vi "LEBITVacuum.CreateLogFile.vi"(0 "i ref in":refnum<vi>, 2 "i attribute in":T1={"setValuePLC"=[], "nickNames"=[], "setValuePLCServiceID"=[], "monValuePLC"=[], "SetValueServiceID"=[], "MonValueServiceID"=[], "SetValue"=[], "AllPLCValues"=[], "CondSpecial2DArray"=[], "CondSpecialIndex"=[], "ReasonForLocking"="", "ReasonForLockingID"=0, "enableValuePLC"=[], "OverwriteCloseSafetyPLC"=[], "OverwriteOpenSafetyPLC"=[], "OverwriteCloseSafetyPLCServiceID"=[], "OverwriteOpenSafetyPLCServiceID"=[], "MKS Address Array"=[], "MKS MeasurementServiceID"=[], "MKS Measurement"=[], "CRYO Measurement"=[], "CRYO MeasurementServiceID"=[], "Special"=[], "Start Date"="", "MKS VISA resource"="COM13", "CRYO VISA resource"="COM13"}, 3 "nickName":string, 4 "value":i16, 5 "error in":errorcluster) -> (14 "i ref out":refnum<vi>, 16 "i attribute out":T1={"setValuePLC"=[], "nickNames"=[], "setValuePLCServiceID"=[], "monValuePLC"=[], "SetValueServiceID"=[], "MonValueServiceID"=[], "SetValue"=[], "AllPLCValues"=[], "CondSpecial2DArray"=[], "CondSpecialIndex"=[], "ReasonForLocking"="", "ReasonForLockingID"=0, "enableValuePLC"=[], "OverwriteCloseSafetyPLC"=[], "OverwriteOpenSafetyPLC"=[], "OverwriteCloseSafetyPLCServiceID"=[], "OverwriteOpenSafetyPLCServiceID"=[], "MKS Address Array"=[], "MKS MeasurementServiceID"=[], "MKS Measurement"=[], "CRYO Measurement"=[], "CRYO MeasurementServiceID"=[], "Special"=[], "Start Date"="", "MKS VISA resource"="COM13", "CRYO VISA resource"="COM13"}, 19 "error out":errorcluster)   [LabVIEW 2014, in "LEBITVacuum.lvlib"]
uses:
  LEBITVacuum.lvlib
  LEBITVacuum.i attribute.ctl
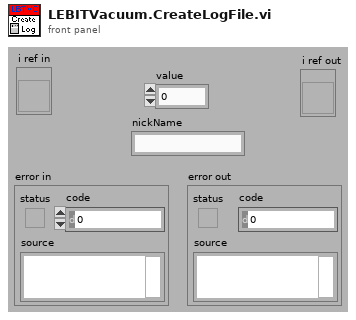
[diagram p1: front panel]
types:
  T1 = typedef "LEBITVacuum.lvlib/LEBITVacuum.i attribute.ctl" = cluster{"setValuePLC":string[], "nickNames":string[], "setValuePLCServiceID":i32[], "monValuePLC":string[], "SetValueServiceID":i32[], "MonValueServiceID":i32[], "SetValue":i16[], "AllPLCValues":string[], "CondSpecial2DArray":string[][], "CondSpecialIndex":i32[], "ReasonForLocking":string, "ReasonForLockingID":i32, "enableValuePLC":string[], "OverwriteCloseSafetyPLC":string[], "OverwriteOpenSafetyPLC":string[], "OverwriteCloseSafetyPLCServiceID":i32[], "OverwriteOpenSafetyPLCServiceID":i32[], "MKS Address Array":i32[][], "MKS MeasurementServiceID":i32[], "MKS Measurement":string[], "CRYO Measurement":string[][], "CRYO MeasurementServiceID":i32[], "Special":string[], "Start Date":string, "MKS VISA resource":refnum<visa-resource-name>, "CRYO VISA resource":refnum<visa-resource-name>}
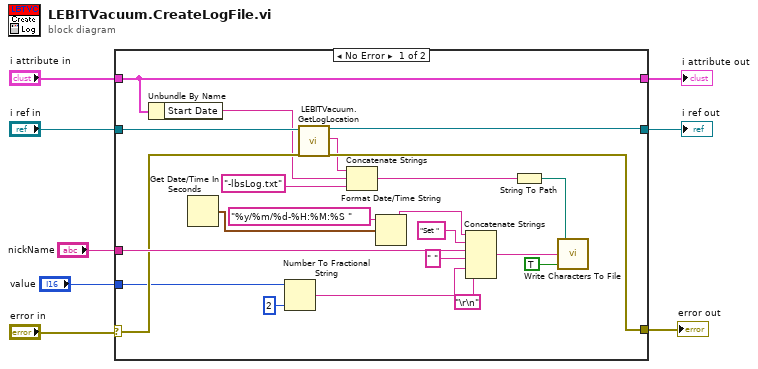
[diagram p0: block diagram]
diagram:
  n1 = case shown="No Error" "error in" {
    selector: "error in" -> [w27 w33]
    tunnel: "nickName" -> [w30 _]
    tunnel: [w26 w33] -> w6
    tunnel: "i ref in" -> [w29 w32]
    tunnel: [w28 w32] -> w2
    tunnel: "i attribute in" -> [w10 w31]
    tunnel: [w10 w31] -> w4
    tunnel: "value" -> [w25 _]
    frame No Error {
      n2 = Unbundle By Name(w10) -> ("Start Date"=w9:string)
      n3 = Get Date/Time In Seconds() -> (seconds since 1Jan1904=w12:timestamp)
      n4 = Number To Fractional String(number=w25, precision (6)=i16 2) -> (F-format string=w15:string)  [unwired: 2 in]
      n5 = call "LEBITVacuum.GetLogLocation.vi"("i ref in"=w29, "error in (no error)"=w27) -> ("i ref out"=w28:refnum<vi>, "log location"=w17:string, "error out 2"=w26:errorcluster)  [unwired: 15 in]
      n6 = Concatenate Strings(w17, w9, "-lbsLog.txt" ("time format string (%c)")) -> (w18:string)
      n7 = Format Date/Time String(time format string (%c)="%y/%m/%d-%H:%M:%S ", seconds (now)=w12) -> (date/time string=w13:string)  [unwired: 1 in]
      n8 = Concatenate Strings(w13, "Set ", w30, " " ("string"), w15, "\r\n") -> (w22:string)
      n9 = String To Path(string=w18) -> (path=w24:path)
      n10 = call <vilib>:"Write Characters To File.vi"("append to file? (new file:F)"=TRUE, "character string"=w22, "file path (dialog if empty)"=w24) -> ()  [unwired: 2 in, 1 out]
    }
    frame Error {
    }
  }
  "error out" <- w6
  "i ref out" <- w2
  "i attribute out" <- w4
